vi "CRYGetPost Pro_all data.vi"(0 "No.VI":i32) -> (1 "Curve array":T1 {"Z data" items=["dB", "Lin"]; "X data" items=["dB", "Lin"]; "Y data" items=["dB", "Lin"]; "Z dB ref" format="%.1f"; "Z axis" items=["Log", "Lin"]; "X dB ref" format="%.1f"; "X axis" items=["Log", "Lin"]; "Y axis" items=["Log", "Lin"]; "Y dB ref" format="%.1f"; "Curve"."z" format="%.2f"; "Curve"."y" format="%.2f"; "Curve"."x" format="%.2f"}, 2 "Value array":T1 {"Z data" items=["dB", "Lin"]; "X data" items=["dB", "Lin"]; "Y data" items=["dB", "Lin"]; "Z dB ref" format="%.1f"; "Z axis" items=["Log", "Lin"]; "X dB ref" format="%.1f"; "X axis" items=["Log", "Lin"]; "Y axis" items=["Log", "Lin"]; "Y dB ref" format="%.1f"; "Curve"."z" format="%.2f"; "Curve"."y" format="%.2f"; "Curve"."x" format="%.2f"}, 3 "Wave array":enum16{"Curves", "Values", "Results", "WFM"}[](array[ring]), 4 "C&W Type array":enum16{"Curves", "Values", "Results", "WFM"}[](array[ring]), 6 "All Names":string[](array[string]), 8 "C&W Names":string[](array[string]), 10 "Value Names":string[](array[string]), 12 "Waveform Array":T3 {"Y dB ref" format="%.1f"; "Y axis" items=["Log", "Lin"]; "Y data" items=["dB", "Lin"]; "X data" items=["dB", "Lin"]}, 13 "Curve Names":string[](array[string]), 14 "Type array":enum16{"Curves", "Values", "Results", "WFM"}[](array[ring]), 15 "Wave names":string[](array[string]))   [LabVIEW 2013]
uses:
  Typedef Control/CRYWaveform Cluster Array.ctl
  Typedef Control/CRYWaveform Cluster.ctl
  Typedef Control/CRYData Cluster Array.ctl
  Typedef Control/CRYData Cluster.ctl
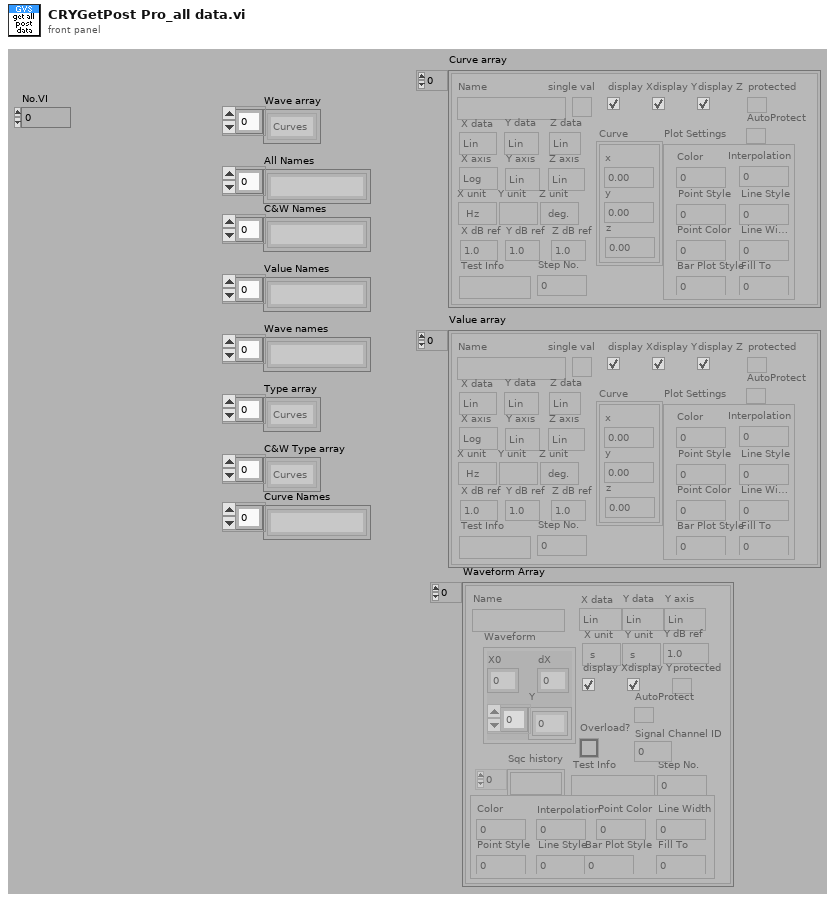
[diagram p1: front panel]
types:
  T1 = typedef "CRYData Cluster Array.ctl" = T2[]
  T2 = typedef "CRYData Cluster.ctl" = cluster{"Name":string, "Curve":cluster{"x":dbl, "y":dbl, "z":dbl}[], "X data":u16, "Y data":u16, "Z data":u16, "X axis":u16, "Y axis":u16, "Z axis":u16, "X unit":string, "Y unit":string, "Z unit":string, "X dB ref":dbl, "Y dB ref":dbl, "Z dB ref":dbl, "single val":bool, "protected":bool, "display X":bool, "display Y":bool, "display Z":bool, "Test Info":string, "Step No.":i32, "Plot Settings":cluster{"Color":u32, "Interpolation":u8, "Point Style":u8, "Line Style":u8, "Point Color":u32, "Line Width":u8, "Bar Plot Style":u8, "Fill To":i16}, "AutoProtect":bool}
  T3 = typedef "CRYWaveform Cluster Array.ctl" = T4[]
  T4 = typedef "CRYWaveform Cluster.ctl" = cluster{"Waveform":cluster{"X0":dbl, "dX":dbl, "Y":sgl[]}, "X data":u16, "Y data":u16, "Y axis":u16, "X unit":string, "Y unit":string, "Y dB ref":dbl, "display Y":bool, "display X":bool, "Overload?":bool, "Test Info":string, "Step No.":i32, "Name":string, "protected":bool, "Sqc history":string[], "Signal Channel ID":i32, "Plot Settings":cluster{"Color":u32, "Interpolation":u8, "Point Style":u8, "Line Style":u8, "Point Color":u32, "Line Width":u8, "Bar Plot Style":u8, "Fill To":i16}, "AutoProtect":bool}
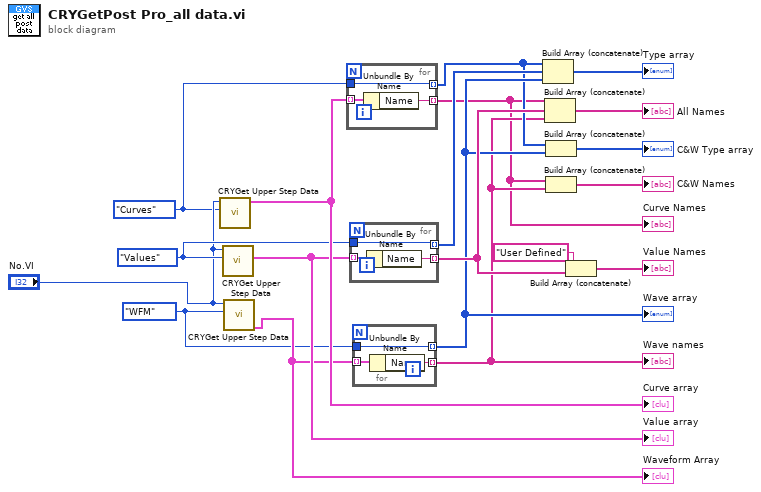
[diagram p0: block diagram]
diagram:
  w11 = enum16{"Curves", "Values", "Results", "WFM"}."Curves" ("Type In")
  w14 = enum16{"Curves", "Values", "Results", "WFM"}."Values" ("Type In")
  w13 = enum16{"Curves", "Values", "Results", "WFM"}."WFM" ("Type In")
  n1 = call "CRYGet Upper Step Data.vi"("Type In"=w11, "No.VI"="No.VI") -> ("Curve array"=w19:T1)  [unwired: 9 out]
  "Curve array" <- w19
  n2 = call "CRYGet Upper Step Data.vi"("Type In"=w14, "No.VI"="No.VI") -> ("Value array"=w18:T1)  [unwired: 9 out]
  "Value array" <- w18
  n3 = call "CRYGet Upper Step Data.vi"("Type In"=w13, "No.VI"="No.VI") -> ("Waveform Array"=w17:T3)  [unwired: 9 out]
  "Waveform Array" <- w17
  n4 = for {
    tunnel: w19 -> [w22] mode=indexing
    tunnel: w11 -> [w21]
    tunnel: [w21] -> w5 mode=indexing
    tunnel: [w20] -> w2 mode=indexing
    n5 = Unbundle By Name(w22) -> ("Name"=w20:string)
  }
  "Curve Names" <- w2
  n6 = for {
    tunnel: w18 -> [w25] mode=indexing
    tunnel: [w24] -> w8 mode=indexing
    tunnel: w14 -> [w23]
    tunnel: [w23] -> w10 mode=indexing
    n7 = Unbundle By Name(w25) -> ("Name"=w24:string)
  }
  n8 = for {
    tunnel: w17 -> [w28] mode=indexing
    tunnel: [w27] -> w3 mode=indexing
    tunnel: w13 -> [w26]
    tunnel: [w26] -> w6 mode=indexing
    n9 = Unbundle By Name(w28) -> ("Name"=w27:string)
  }
  "Wave names" <- w3
  "Wave array" <- w6
  n10 = Build Array (concatenate)(w5, w10, w6) -> (→"Type array":enum16{"Curves", "Values", "Results", "WFM"}[])
  n11 = Build Array (concatenate)(w2, w8, w3) -> (→"All Names":string[])
  n12 = Build Array (concatenate)(w5, w6) -> (→"C&W Type array":enum16{"Curves", "Values", "Results", "WFM"}[])
  n13 = Build Array (concatenate)(w2, w3) -> (→"C&W Names":string[])
  n14 = Build Array (concatenate)("User Defined", w8) -> (→"Value Names":string[])
